vi "LV Paint.vi"() -> ()   [LabVIEW 2020, in "examples.lvlib"]
doc: "Demonstrate using the LabVIEW Picture Indicator for interactive operations on Images and the utility VIs included with this toolkit for scalling and drawing Images and working with LabVIEW Picture Indicator and Image Co-ordinate Systems."
uses:
  examples.lvlib
  common/Image Size (Integer).ctl
  <vilib>/event_ctls.llb/sizeaction.ctl
  image/ARGB Colour.ctl
  <vilib>/Utility/sysdir.llb/System Directory Type.ctl
  image/New Image (ARGB Preallocated).vi
  image/Draw Image to Picture (ARGB).vi
  image/Size (ARGB).vi
  image/Draw Circle (ARGB).vi
  image/Write Image File (ARGB).vi
  image/New Image (ARGB Preallocated).vi/3321fa97-f432-4e1e-8db9-a0df79aed21b.vi
  image/ARGB Colour to U32 Pixel Value.vi
  image/Draw Image to Picture (ARGB).vi/8cd07b1b-062e-4fe4-9e87-2eb3dc89fe0e.vi
  image/Size (ARGB).vi/69a1505b-b287-44ed-9ef9-f10ed7b260f4.vi
  image/Draw Circle (ARGB).vi/8336a1cf-e433-4bea-8080-376bdb783d4e.vi
  image/Write Image File (ARGB).vi/9723f547-2605-4a38-b7b5-a8bc0a93fff0.vi
  <vilib>/Utility/error.llb/Error Cluster From Error Code.vi
  image/image.lvlib
  common/common.lvlib
panel:
  in  "Size":u8=15 min=3
  in  "Colour":u32(colorbox)=16448250
  out "Picture":picture
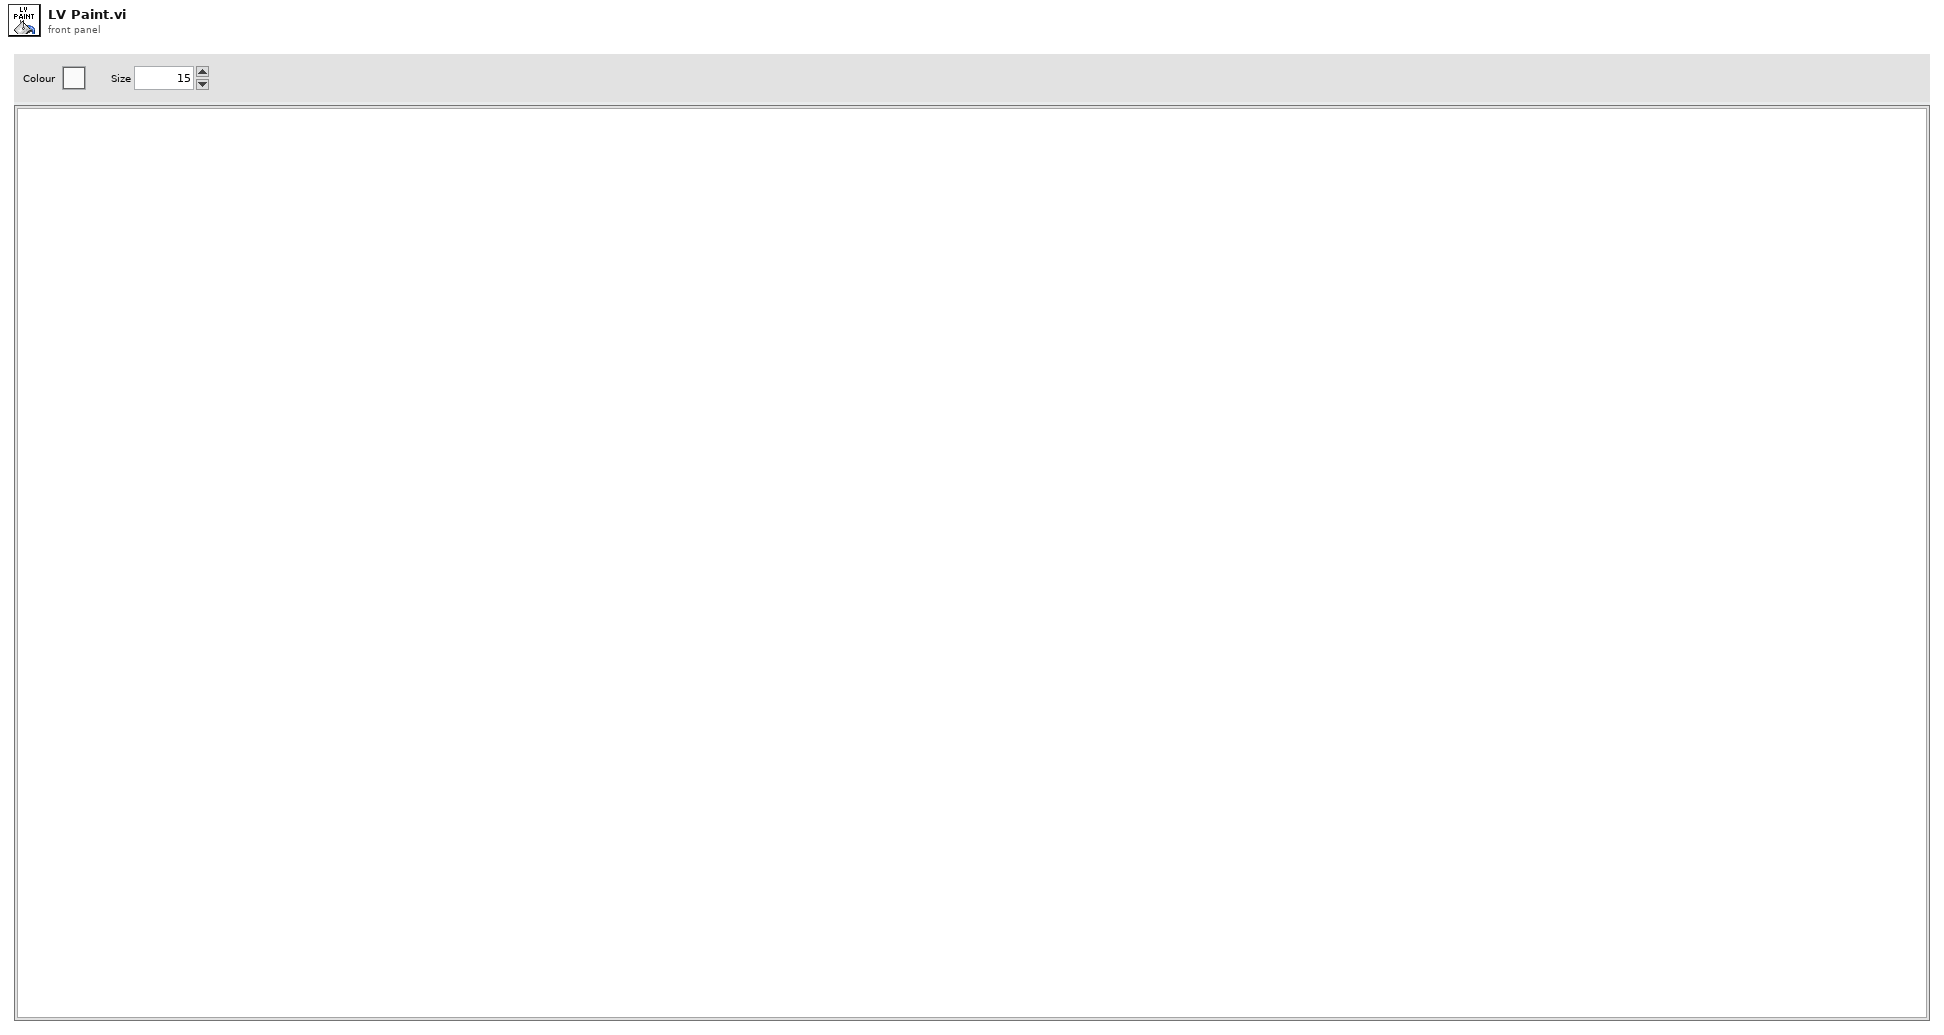
[diagram p1: front panel]
types:
  T1 = typedef "common.lvlib/Image Size (Integer).ctl" = cluster{"Width":u16, "Height":u16}
  T2 = typedef "image.lvlib/ARGB Image.ctl" = refnum<data-value>
  T3 = typedef "image.lvlib/Image Draw Offset.ctl" = cluster{"Left":i16, "Top":i16}
  T4 = typedef "sizeaction.ctl" = enum32{"Minimized", "Maximized", "Resized"}
  T5 = typedef "image.lvlib/ARGB Colour.ctl" = cluster{"Alpha":u8, "RGB":u32}
  T6 = typedef "LVRectTypeDef.ctl" = cluster{"Left":i16, "Top":i16, "Right":i16, "Bottom":i16}
  T7 = typedef "LVPoint32TypeDef.ctl" = cluster{"Horizontal":i32, "Vertical":i32}
  T8 = typedef "common.lvlib/Image Point (Float).ctl" = cluster{"x":dbl, "y":dbl}
  T9 = typedef "System Directory Type.ctl" = i32
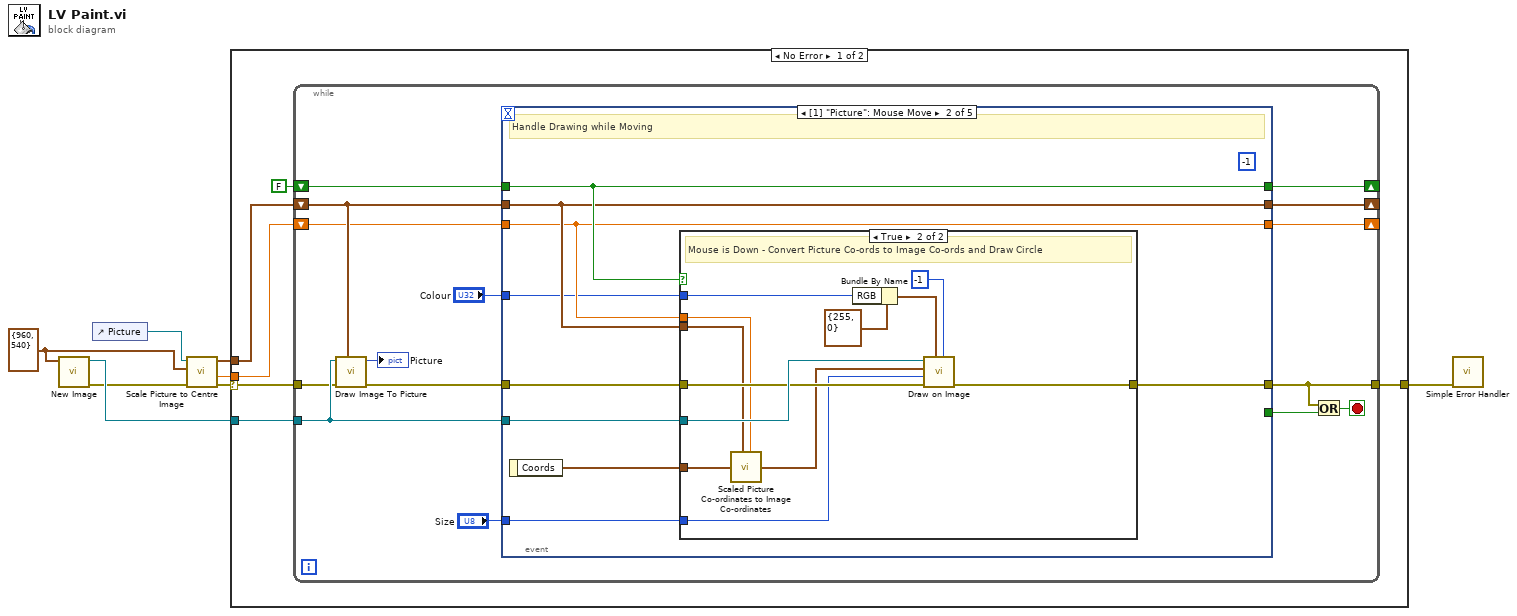
[diagram p0: block diagram]
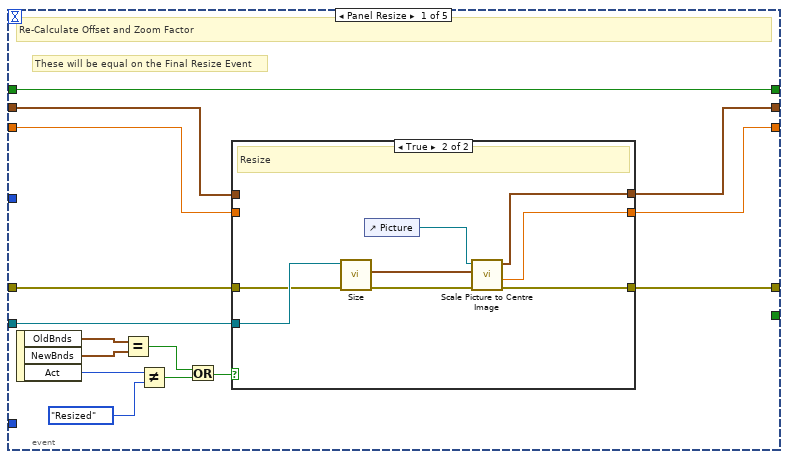
[diagram p2: hidden frame]
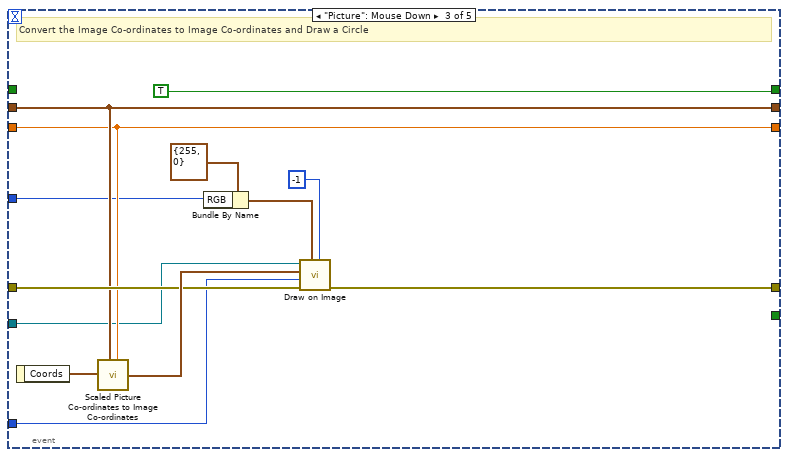
[diagram p5: hidden frame]
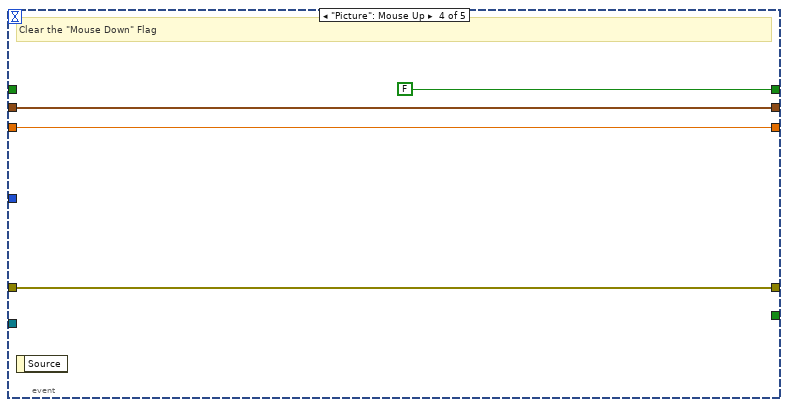
[diagram p6: hidden frame]
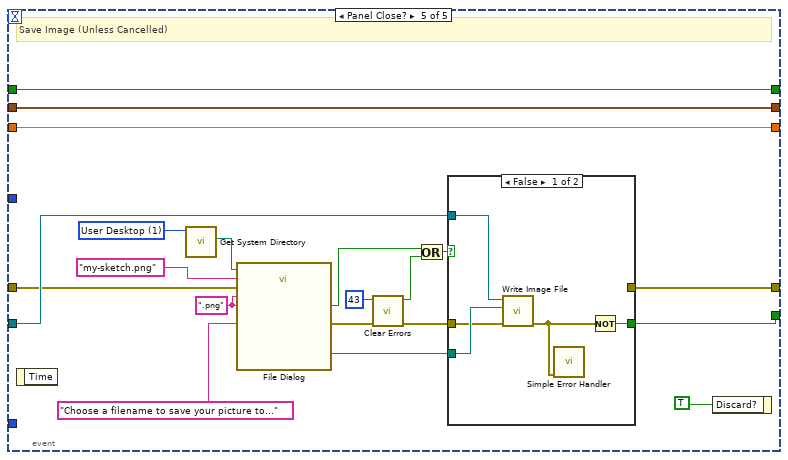
[diagram p7: hidden frame]
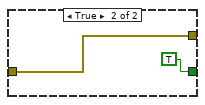
[diagram p8: hidden frame]
diagram:
  w3 = T1 {"Width"=960, "Height"=540} ("Preallocated Image Size (Default: 0,0)")
  n1 = call-poly "New Image.vi"("Preallocated Image Size (Default: 0,0)"=w3) -> ("error out"=w6:errorcluster, "ARGB Image"=w8:T2)  [unwired: 9 in]
  n2 = control-ref of="Picture"() -> (w7:refnum<vi>)
  n3 = call "Scale Picture to Centre Image.vi"("error in (no error)"=w6, "Image Size"=w3, "Picture in"=w7) -> ("error out"=w5:errorcluster, "Zoom Factor Set"=w2:dbl, "Draw Image to Picture Offset"=w4:T3)  [unwired: 6 in]
  n4 = case shown="No Error" w5 {
    selector: w5 -> [w13 w122]
    tunnel: w8 -> [w14 _]
    tunnel: w4 -> [w12 _]
    tunnel: w2 -> [w11 _]
    tunnel: [w9 w122] -> w1
    frame No Error {
      n5 = while {
        tunnel: w14 -> [w28]
        tunnel: w13 -> [w27]
        shift-right: [w25] -> _
        shift-left: w12 -> [w26]
        shift-right: [w20] -> _
        shift-left: w11 -> [w21]
        shift-right: [w19] -> _
        shift-left: FALSE -> [w18]
        tunnel: [w15] -> w9
        stop <- w22 stop-if-true
        n6 = call-poly "Draw Image To Picture.vi"("Image Draw Offset (Default 0,0)"=w26, "error in (no error)"=w27, "ARGB Image Source in"=w28) -> ("error out"=w23:errorcluster, "Picture"=→"Picture":picture)  [unwired: 7 in]
        n7 = event shown="[1] \"Picture\": Mouse Move" {
          selector: _ -> [_ _ _ _ _]
          dyn-events: _ -> [_ _ _ _ _]
          timeout: _ -> [_ _ _ _ _]
          tunnel: w28 -> [w44 w62 w78 _ w107]
          tunnel: [_ _ _ _ w104] -> w29
          tunnel: w26 -> [w35 w59 w82 w94 w106]
          tunnel: [w42 w59 w82 w94 w106] -> w25
          tunnel: w23 -> [w43 w61 w85 w91 w105]
          tunnel: [w41 w60 w84 w91 w103] -> w15
          tunnel: w21 -> [w34 w58 w81 w93 w102]
          tunnel: [w40 w58 w81 w93 w102] -> w20
          tunnel: [w39 w64 TRUE FALSE w101] -> w19
          tunnel: w18 -> [w39 w64 _ _ w101]
          tunnel: "Colour" -> [_ w57 w80 _ _]
          tunnel: "Size" -> [_ w56 w79 _ _]
          event Panel Resize {
            # "These will be equal on the Final Resize Event"
            # "Re-Calculate Offset and Zoom Factor"
            n8 = event-data() -> ("OldBnds"=w38:T6, "NewBnds"=w37:T6, "Act"=w32:T4)  [unwired: 1 in]
            n9 = Equal?(x=w38, y=w37) -> (x = y?=w36:bool)
            n10 = Not Equal?(x=w32, y=sizeaction."Resized") -> (x != y?=w30:bool)
            n11 = Or(x=w36, y=w30) -> (x .or. y?=w33:bool)
            n12 = case shown="True" w33 {
              tunnel: w44 -> [_ w54]
              tunnel: w43 -> [w45 w53]
              tunnel: [w47 w50] -> w42
              tunnel: [w45 w49] -> w41
              tunnel: [w46 w48] -> w40
              tunnel: w35 -> [w47 _]
              tunnel: w34 -> [w46 _]
              frame False {
                # "Don't Resize"
              }
              frame True {
                # "Resize"
                n13 = call-poly "Size.vi"("error in (no error)"=w53, "ARGB Image in"=w54) -> ("error out"=w52:errorcluster, "Image Size"=w51:T1)  [unwired: 7 in, 1 out]
                n14 = control-ref of="Picture"() -> (w55:refnum<vi>)
                n15 = call "Scale Picture to Centre Image.vi"("error in (no error)"=w52, "Image Size"=w51, "Picture in"=w55) -> ("error out"=w49:errorcluster, "Zoom Factor Set"=w48:dbl, "Draw Image to Picture Offset"=w50:T3)  [unwired: 6 in]
              }
            }
          }
          event "Picture": Mouse Move {
            (unwired) -1
            # "Handle Drawing while Moving"
            n16 = event-data() -> ("Coords"=w63:T7)  [unwired: 1 in]
            n17 = case shown="True" w64 {
              tunnel: w63 -> [_ w71]
              tunnel: w62 -> [_ w77]
              tunnel: w61 -> [w65 w74]
              tunnel: [w65 w73] -> w60
              tunnel: w59 -> [_ w70]
              tunnel: w58 -> [_ w69]
              tunnel: w57 -> [_ w67]
              tunnel: w56 -> [_ w66]
              frame False {
                # "Mouse Not Down"
              }
              frame True {
                # "Mouse is Down - Convert Picture Co-ords to Image Co-ords and Draw Circle"
                n18 = call "Scaled Picture Co-ordinates to Image Co-ordinates.vi"("Image Draw Offset"=w70, "Picture Control Coords"=w71, "Zoom Factor Set"=w69) -> ("Image Point"=w68:T8)  [unwired: 6 in]
                n19 = Bundle By Name(cluster=T5 {"Alpha"=255, "RGB"=0} ("ARGB Colour"), "RGB"=w67) -> (w75:T5)
                n20 = call-poly "Draw on Image.vi"("Thickness (Default: 1)"=-1, "ARGB Colour"=w75, "error in (no error)"=w74, "Radius"=w66, "Centre"=w68, "ARGB Image in"=w77) -> ("error out"=w73:errorcluster)  [unwired: 4 in, 1 out]
              }
            }
          }
          event "Picture": Mouse Down {
            # "Convert the Image Co-ordinates to Image Co-ordinates and Draw a Circle"
            n21 = event-data() -> ("Coords"=w83:T7)  [unwired: 1 in]
            n22 = call "Scaled Picture Co-ordinates to Image Co-ordinates.vi"("Image Draw Offset"=w82, "Picture Control Coords"=w83, "Zoom Factor Set"=w81) -> ("Image Point"=w86:T8)  [unwired: 6 in]
            n23 = Bundle By Name(cluster=T5 {"Alpha"=255, "RGB"=0} ("ARGB Colour"), "RGB"=w80) -> (w88:T5)
            n24 = call-poly "Draw on Image.vi"("Thickness (Default: 1)"=-1, "ARGB Colour"=w88, "error in (no error)"=w85, "Radius"=w79, "Centre"=w86, "ARGB Image in"=w78) -> ("error out"=w84:errorcluster)  [unwired: 4 in, 1 out]
          }
          event "Picture": Mouse Up {
            # "Clear the \"Mouse Down\" Flag"
            n25 = event-data() -> ()  [unwired: 1 in, 1 out]
          }
          event Panel Close? {
            w100 = ".png" ("pattern label")
            w112 = T9 1 items=["User Home"=0, "User Desktop"=1, "User Documents"=2, "User Application Data"=3, "User Preferences"=4, "User Temporary"=5, "Public Documents"=6, "Public Application Data"=7, "Public Preferences"=8, "Public Cache"=13, "System Core Libraries"=9, "System Installed Libraries"=10, "Application Files"=11, "Boot Volume Root"=12] ("system directory type")
            # "Save Image (Unless Cancelled)"
            n26 = event-data() -> ()  [unwired: 1 in, 1 out]
            n27 = call <vilib>:"Get System Directory.vi"("system directory type"=w112) -> ("system directory"=w113:path)  [unwired: 10 in]
            n28 = call "File Dialog"("start path"=w113, "prompt"="Choose a filename to save your picture to...", "default name"="my-sketch.png", "error in"=w105, "pattern (all files)"=w100, "pattern label"=w100) -> ("selected path"=w108:path, "cancelled"=w109:bool, "error out"=w99:errorcluster)  [unwired: 6 in, 1 out]
            n29 = call <vilib>:"Clear Errors.vi"("error in (no error)"=w99, "specific error code to clear (0: all)"=43) -> ("error out"=w98:errorcluster, "specific error cleared?"=w96:bool)  [unwired: 4 in]
            n30 = Or(x=w109, y=w96) -> (x .or. y?=w97:bool)
            n31 = case shown="False" w97 {
              tunnel: w108 -> [w119 _]
              tunnel: w107 -> [w118 _]
              tunnel: [_ w121] -> w103
              tunnel: w98 -> [w117 w121]
              tunnel: [w116 TRUE] -> w104
              frame False {
                n32 = call-poly "Write Image File.vi"("error in (no error)"=w117, "Filepath in"=w119, "ARGB Image Source in"=w118) -> ("error out"=w115:errorcluster)  [unwired: 7 in, 1 out]
                n33 = call <vilib>:"Simple Error Handler.vi"("error in (no error)"=w115) -> ()  [unwired: 4 in, 5 out]
                n34 = Not(x=w115) -> (.not. x?=w116:bool)
              }
              frame True {
              }
            }
            n35 = event-data("Discard?"=TRUE) -> ()  [unwired: 1 in, 1 out]
          }
        }
        n36 = Or(x=w15, y=w29) -> (x .or. y?=w22:bool)
      }
    }
    frame Error {
    }
  }
  n37 = call <vilib>:"Simple Error Handler.vi"("error in (no error)"=w1) -> ()  [unwired: 4 in, 5 out]
